vi "Get servicio from ui.vi"(8 "error in (no error)":errorcluster, 10 "Servicio seleccionado":string, 11 "Contabilidad in":refnum<class "Contabilidad.lvclass">) -> (0 "error out":errorcluster, 3 "Contabilidad out":refnum<class "Contabilidad.lvclass">)   [LabVIEW 2020, in "Contabilidad.lvlib" / "Contabilidad.lvclass"]
uses:
  Contabilidad.lvclass
  Contabilidad.lvclass/Contabilidad.ctl
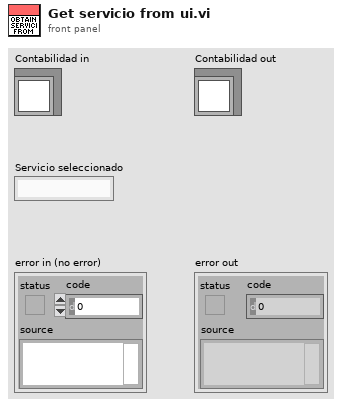
[diagram p1: front panel]
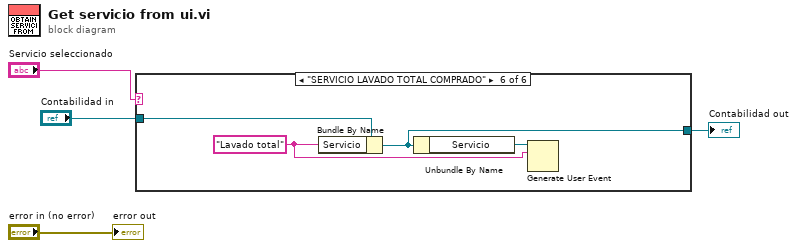
[diagram p0: block diagram]
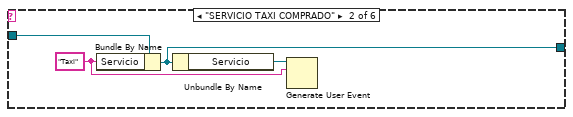
[diagram p3: hidden frame]
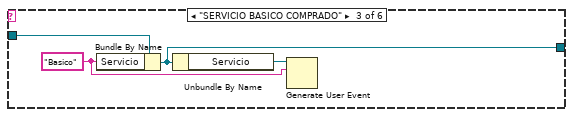
[diagram p4: hidden frame]
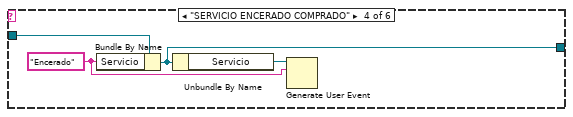
[diagram p5: hidden frame]
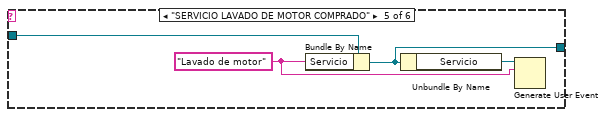
[diagram p6: hidden frame]
diagram:
  n1 = case shown="\"SERVICIO LAVADO TOTAL COMPRADO\"" "Servicio seleccionado" {
    tunnel: "Contabilidad in" -> [_ w8 w12 w16 w20 w24]
    tunnel: [_ w5 w9 w13 w17 w21] -> w1
    frame Default {
    }
    frame "SERVICIO TAXI COMPRADO" {
      w6 = "Taxi" ("Servicio")
      n2 = Bundle By Name(cluster=w8, "Servicio"=w6) -> (w5:refnum<class "Contabilidad.lvclass">)
      n3 = Unbundle By Name(w5) -> ("Servicio"=w7:refnum<user-event>)
      n4 = Generate User Event(user event=w7, event data cluster=w6) -> ()  [unwired: 2 in, 2 out]
    }
    frame "SERVICIO BASICO COMPRADO" {
      w10 = "Basico" ("Servicio")
      n5 = Bundle By Name(cluster=w12, "Servicio"=w10) -> (w9:refnum<class "Contabilidad.lvclass">)
      n6 = Unbundle By Name(w9) -> ("Servicio"=w11:refnum<user-event>)
      n7 = Generate User Event(user event=w11, event data cluster=w10) -> ()  [unwired: 2 in, 2 out]
    }
    frame "SERVICIO ENCERADO COMPRADO" {
      w14 = "Encerado" ("Servicio")
      n8 = Bundle By Name(cluster=w16, "Servicio"=w14) -> (w13:refnum<class "Contabilidad.lvclass">)
      n9 = Unbundle By Name(w13) -> ("Servicio"=w15:refnum<user-event>)
      n10 = Generate User Event(user event=w15, event data cluster=w14) -> ()  [unwired: 2 in, 2 out]
    }
    frame "SERVICIO LAVADO DE MOTOR COMPRADO" {
      w18 = "Lavado de motor" ("Servicio")
      n11 = Bundle By Name(cluster=w20, "Servicio"=w18) -> (w17:refnum<class "Contabilidad.lvclass">)
      n12 = Unbundle By Name(w17) -> ("Servicio"=w19:refnum<user-event>)
      n13 = Generate User Event(user event=w19, event data cluster=w18) -> ()  [unwired: 2 in, 2 out]
    }
    frame "SERVICIO LAVADO TOTAL COMPRADO" {
      w22 = "Lavado total" ("Servicio")
      n14 = Bundle By Name(cluster=w24, "Servicio"=w22) -> (w21:refnum<class "Contabilidad.lvclass">)
      n15 = Unbundle By Name(w21) -> ("Servicio"=w23:refnum<user-event>)
      n16 = Generate User Event(user event=w23, event data cluster=w22) -> ()  [unwired: 2 in, 2 out]
    }
  }
  "Contabilidad out" <- w1
  "error out" <- "error in (no error)"
